vi "osd_send_data_Len_parse.vi"(10 "bypara":u8, 11 "bySubcmd":u8) -> (3 "byDataLen":u8)   [LabVIEW 2016]
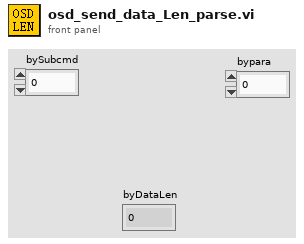
[diagram p1: front panel]
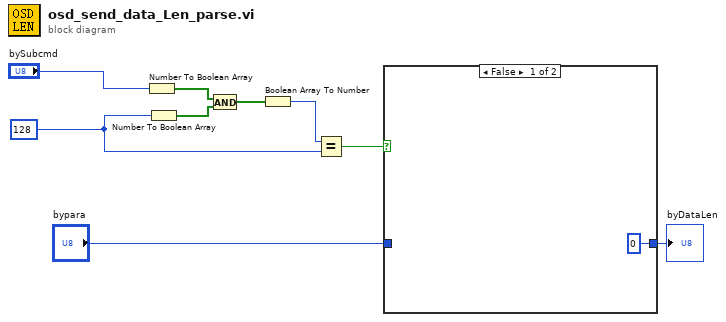
[diagram p0: block diagram]
diagram:
  w4 = u8 128 ("number")
  n1 = Number To Boolean Array(number="bySubcmd") -> (Boolean array=w8:bool[])
  n2 = Number To Boolean Array(number=w4) -> (Boolean array=w7:bool[])
  n3 = And(x=w8, y=w7) -> (x .and. y?=w6:bool[])
  n4 = Boolean Array To Number(Boolean array=w6) -> (number=w5:u8)
  n5 = Equal?(x=w5, y=w4) -> (x = y?=w3:bool)
  n6 = case shown="False" w3 {
    tunnel: "bypara" -> [_ w11]
    tunnel: [u8 0 ("bypara") w11] -> w1
    frame False {
    }
    frame True {
    }
  }
  "byDataLen" <- w1
